vi "MakeMatlabExperiment.vi"(8 "error in":errorcluster, 11 "experimentFilepath":path) -> (0 "error out":errorcluster, 1 "erros?":bool, 2 "errors":string, 3 "ExpID":string)   [LabVIEW 2017]
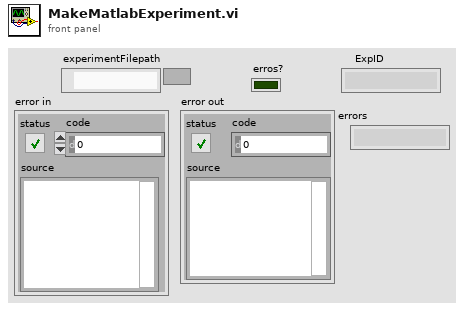
[diagram p1: front panel]
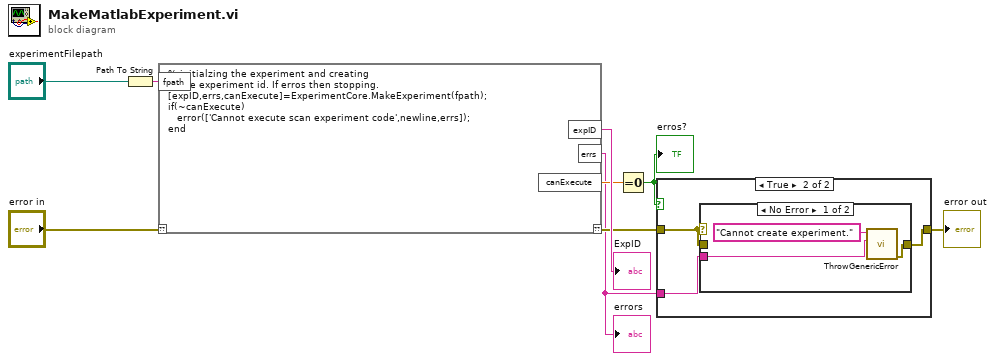
[diagram p0: block diagram]
diagram:
  n1 = Path To String(path="experimentFilepath") -> (string=w8:string)
  n2 = script code="% initialzing the experiment and creating\n% the experiment id. If erros then stopping.\n[expID,errs,canExecute]=ExperimentCore.MakeExperiment(fpath);\nif(~canExecute)\n   error(['Cannot execute scan experiment code',newline,errs]);\nend"("??"="error in", "fpath"=w8) -> ("??"=w4:errorcluster, "expID"=→"ExpID":string, "errs"=w2:string, "canExecute"=w6:dbl)
  "errors" <- w2
  n3 = Equal To 0?(x=w6) -> (x = 0?=w1:bool)
  "erros?" <- w1
  n4 = case shown="True" w1 {
    tunnel: w4 -> [w10 w11]
    tunnel: [w10 w12] -> w3
    tunnel: w2 -> [_ w13]
    frame False {
    }
    frame True {
      n5 = case shown="No Error" w11 {
        tunnel: w11 -> [_ w17]
        tunnel: w13 -> [w15 _]
        tunnel: [w16 w17] -> w12
        frame No Error {
          n6 = call "ThrowGenericError.vi"("Error info"=w15, "TheError"="Cannot create experiment.") -> ("error out"=w16:errorcluster)  [unwired: 9 in]
        }
        frame Error {
        }
      }
    }
  }
  "error out" <- w3
